vi "ImagenDataReadingStringToClusterFormar.vi"(11 "StringFormat":string[](array[string])) -> (3 "ClusterFormat":T1)   [LabVIEW 2014]
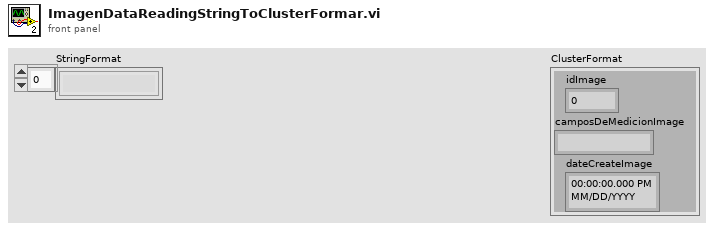
[diagram p1: front panel]
types:
  T1 = cluster{"idImage":dbl, "camposDeMedicionImage":string, "dateCreateImage":timestamp}
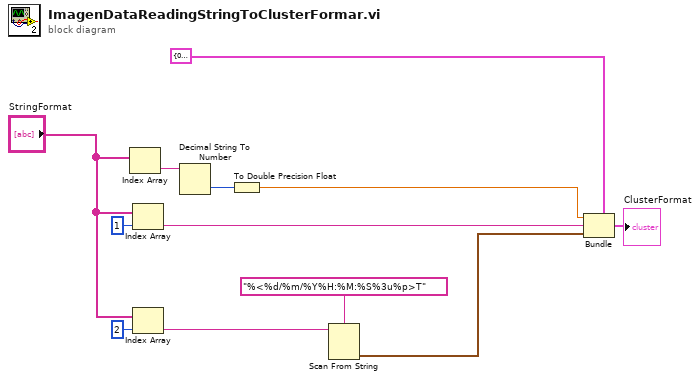
[diagram p0: block diagram]
diagram:
  n1 = Index Array(array="StringFormat") -> (element=w12:string)  [unwired: 1 in]
  n2 = Index Array(array="StringFormat", index=1) -> (element=w7:string)
  n3 = Index Array(array="StringFormat", index=2) -> (element=w2:string)
  n4 = Decimal String To Number(string=w12) -> (number=w9:i32)  [unwired: 2 in, 1 out]
  n5 = To Double Precision Float(number=w9) -> (double precision float=w8:dbl)
  n6 = Scan From String(format string="%<%d/%m/%Y%H:%M:%S%3u%p>T", input string=w2) -> (output 1=w1:timestamp)  [unwired: 3 in, 3 out]
  n7 = Bundle(cluster=T1 {"idImage"=0.0, "camposDeMedicionImage"="", "dateCreateImage"=timestamp(0 s since 1904-01-01)} ("dataToQueryOfRead"), "idImage"=w8, "camposDeMedicionImage"=w7, "dateCreateImage"=w1) -> (→"ClusterFormat":T1)
